vi "FarbeWechseln(SubVI).vi"(9 "Panel Farbe":u32(colorbox), 10 "Panel Farbe 2":u32 format="%06x", 11 "Boolesch":bool) -> (1 "Panel Farbe 3":u32, 2 "Deaktiviert 2":T1(ring), 3 "Deaktiviert":T1(ring))   [LabVIEW 2017]
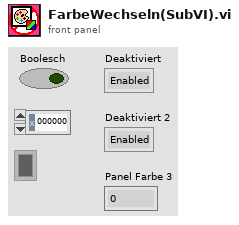
[diagram p1: front panel]
types:
  T1 = enum8{"Enabled", "Disabled", "Disabled and Grayed Out"}
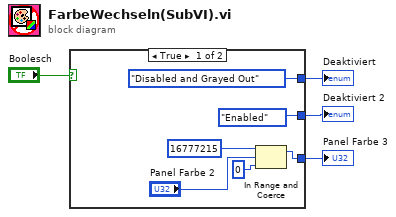
[diagram p0: block diagram]
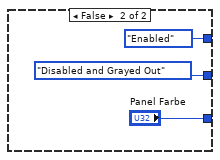
[diagram p2: hidden frame]
diagram:
  n1 = case shown="True" "Boolesch" {
    tunnel: [T1."Enabled" ("Deaktiviert") T1."Disabled and Grayed Out" ("Deaktiviert")] -> w1
    tunnel: [T1."Disabled and Grayed Out" ("Deaktiviert") T1."Enabled" ("Deaktiviert")] -> w3
    tunnel: [w6 "Panel Farbe"] -> w4
    frame True {
      n2 = In Range and Coerce(upper limit=u32 16777215 ("Obergrenze"), x="Panel Farbe 2", lower limit=u32 0 ("Untergrenze")) -> (coerced(x)=w6:u32)  [unwired: 1 out]
    }
    frame False {
    }
  }
  "Panel Farbe 3" <- w4
  "Deaktiviert" <- w3
  "Deaktiviert 2" <- w1
